vi "analyze cpu.vi"(8 "error in (no error)":errorcluster, 10 "offset (0)":i64, 11 "file path":path) -> (0 "error out":errorcluster, 2 "cpu load stats":T1, 3 "data":dbl[](array[numeric]))   [LabVIEW 2014]
uses:
  <vilib>/gmath/statdist.llb/st_Percentiles (scalar).vi
  <vilib>/Analysis/NI_AALBase.lvlib
  <vilib>/gmath/NI_Gmath.lvlib
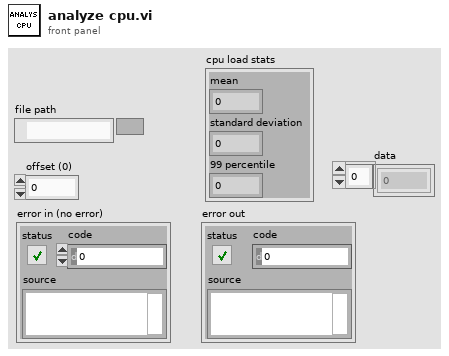
[diagram p1: front panel]
types:
  T1 = cluster{"mean":dbl, "standard deviation":dbl, "99 percentile":dbl}
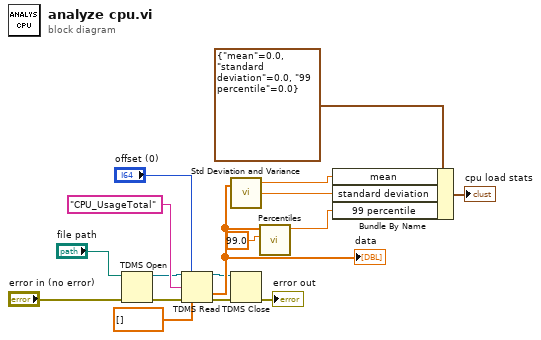
[diagram p0: block diagram]
diagram:
  n1 = TDMS Open(8:"error in (no error)", 11:"file path") -> (0:w1:errorcluster, 3:w2:refnum<k34>)  [unwired: 5 in]
  n2 = TDMS Read(0:w2, 1:"offset (0)", 7:"CPU_UsageTotal" ("channel name(s) in"), 11:w1, 12:dbl[] []) -> (4:w6:refnum<k34>, 10:w9:dbl[], 15:w7:errorcluster)  [unwired: 3 in, 3 out]
  "data" <- w9
  n3 = call <vilib>:"Std Deviation and Variance.vi"("X"=w9) -> ("mean"=w12:dbl, "standard deviation"=w13:dbl)  [unwired: 1 in, 1 out]
  n4 = TDMS Close(8:w7, 11:w6) -> (0:→"error out":errorcluster)  [unwired: 1 out]
  n5 = call-poly <vilib>:"Percentiles.vi"("p"=99.0, "x array"=w9) -> ("percentile"=w14:dbl)  [unwired: 8 in, 1 out]
  n6 = Bundle By Name(cluster=T1 {"mean"=0.0, "standard deviation"=0.0, "99 percentile"=0.0}, "mean"=w12, "standard deviation"=w13, "99 percentile"=w14) -> (→"cpu load stats":T1)
